vi "Auto 8.vi"(8 "Error In":errorcluster) -> (0 "Error Out":errorcluster)   [LabVIEW 2014]
uses:
  <vilib>/Rock Robotics/Network Tables/SD Read Boolean.vi
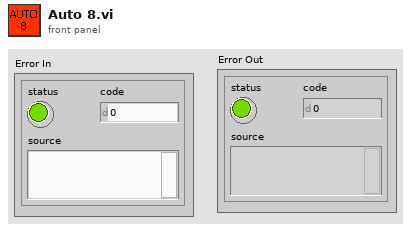
[diagram p1: front panel]
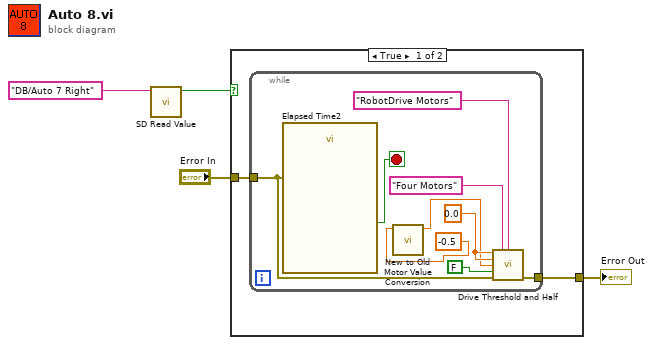
[diagram p0: block diagram]
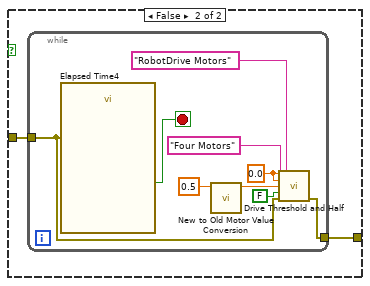
[diagram p2: hidden frame]
diagram:
  n1 = call-poly <vilib>:"SD Read Value.vi"("Name"="DB/Auto 7 Right") -> ("Boolean"=w3:bool)  [unwired: 8 in, 2 out]
  n2 = case shown="True" w3 {
    tunnel: "Error In" -> [w6 w17]
    tunnel: [w5 w16] -> w1
    frame True {
      n3 = while {
        tunnel: w6 -> [w9]
        tunnel: [w11] -> w5
        stop <- w10 stop-if-true
        w12 = 0.0 ("Arm Value")
        n4 = call "Elapsed Time2"("error in (no error)"=w9) -> ("Time has Elapsed"=w10:bool)  [unwired: 11 in, 7 out]
        n5 = call "New to Old Motor Value Conversion.vi"("Motor Value In"=-0.5 ("X In")) -> ("New to Old Conversion Value Out"=w7:dbl)  [unwired: 9 in, 1 out]
        n6 = call "Drive Threshold and Half.vi"("X In"=w12, "Drive refnum name"="Four Motors" ("refnum name"), "Send to DB Name"="RobotDrive Motors" ("Name"), "Y In"=w12, "R In"=w7, "Speed Toggle"=FALSE ("Grabber Open/Close"), "Error In"=w9) -> ("Error Out"=w11:errorcluster)  [unwired: 8 in]
      }
    }
    frame False {
      n7 = while {
        tunnel: w17 -> [w20]
        tunnel: [w23] -> w16
        stop <- w21 stop-if-true
        w22 = 0.0 ("Arm Value")
        n8 = call "Elapsed Time4"("error in (no error)"=w20) -> ("Time has Elapsed"=w21:bool)  [unwired: 11 in, 7 out]
        n9 = call "New to Old Motor Value Conversion.vi"("Motor Value In"=0.5 ("X In")) -> ("New to Old Conversion Value Out"=w18:dbl)  [unwired: 9 in, 1 out]
        n10 = call "Drive Threshold and Half.vi"("X In"=w22, "Drive refnum name"="Four Motors" ("refnum name"), "Send to DB Name"="RobotDrive Motors" ("Name"), "Y In"=w22, "R In"=w18, "Speed Toggle"=FALSE ("Grabber Open/Close"), "Error In"=w20) -> ("Error Out"=w23:errorcluster)  [unwired: 8 in]
      }
    }
  }
  "Error Out" <- w1
